vi "MTM2_getNextSample_rawDisplacement.vi"(8 "error in (no error)":errorcluster, 11 "rawDisplacement_Ctl":T1={"rawPosition[72]"=[0.0, 0.0, 0.0, 0.0, 0.0, 0.0, 0.0, 0.0, 0.0, 0.0, 0.0, 0.0, 0.0, 0.0, 0.0, 0.0, 0.0, 0.0, 0.0, 0.0, 0.0, 0.0, 0.0, 0.0, 0.0, 0.0, 0.0, 0.0, 0.0, 0.0, 0.0, 0.0, 0.0, 0.0, 0.0, 0.0, 0.0, 0.0, 0.0, 0.0, 0.0, 0.0, 0.0, 0.0, 0.0, 0.0, 0.0, 0.0, 0.0, 0.0, 0.0, 0.0, 0.0, 0.0, 0.0, 0.0, 0.0, 0.0, 0.0, 0.0, 0.0, 0.0, 0.0, 0.0, 0.0, 0.0, 0.0, 0.0, 0.0, 0.0, 0.0, 0.0]}) -> (0 "error out":errorcluster, 2 "function return":i32, 3 "rawDisplacement_Ctl out":T1)   [LabVIEW 2018, in "SALLV_MTM2.lvlib"]
doc: "int MTM2_shm_getNextSample_rawDisplacementLV(MTM2_rawDisplacementLV *rawDisplacement_Ctl );"
uses:
  SALLV_MTM2.lvlib
  DataTypes/rawDisplacement.ctl
  SALLV_MTM2.so
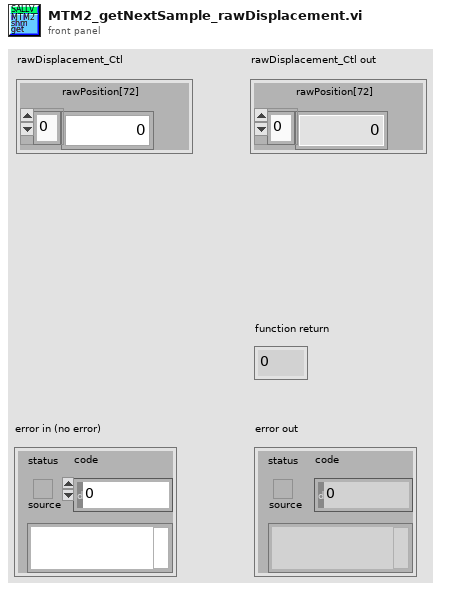
[diagram p1: front panel]
types:
  T1 = typedef "SALLV_MTM2.lvlib/rawDisplacement.ctl" = cluster{"rawPosition[72]":dbl[]}
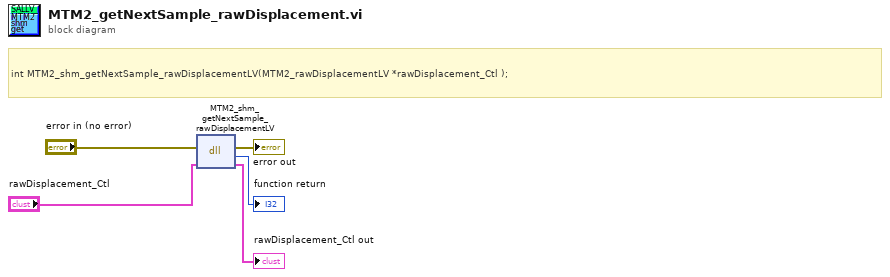
[diagram p0: block diagram]
diagram:
  # "int MTM2_shm_getNextSample_rawDisplacementLV(MTM2_rawDisplacementLV *rawDisplacement_Ctl );"
  n1 = dll-call lib="home/ttsai/Document/salApiMTM2/SALLV_MTM2/SALLV_MTM2.*" fn="MTM2_shm_getNextSample_rawDisplacementLV"(error in="error in (no error)", "rawDisplacement_Ctl"="rawDisplacement_Ctl") -> (error out=→"error out":errorcluster, →"function return":i32, "rawDisplacement_Ctl"=→"rawDisplacement_Ctl out":T1)  [unwired: 2 in, 1 out]
